vi "Splash.vi"(4 "warning sign":refnum<vi>, 5 "Cluster control array":refnum<vi>[](array[refnum])=[refnum, refnum, refnum], 6 "Firmware :":refnum<vi>, 7 "Pressure:":refnum<vi>, 8 "error in (no error)":errorcluster, 10 "Init Ref":T1, 11 "Stop":refnum<vi>) -> (0 "error out":errorcluster)   [LabVIEW 2018]
uses:
  PublicSubVI/Class/FileManager/FM/ctl/_PC_Pub_FM ctrlFileRefnumEnum.ctl
  PublicSubVI/Ctl/RegistyFunc.ctl
  <vilib>/Utility/error.llb/Error Cluster From Error Code.vi
  <vilib>/ErrorRing/Error Ring.xnode
  PublicSubVI/Class/SigInfo/SigInfo.lvclass
  PublicSubVI/Class/Sig2MS/Sig2MS.lvclass
panel:
  out "Status String Display":string
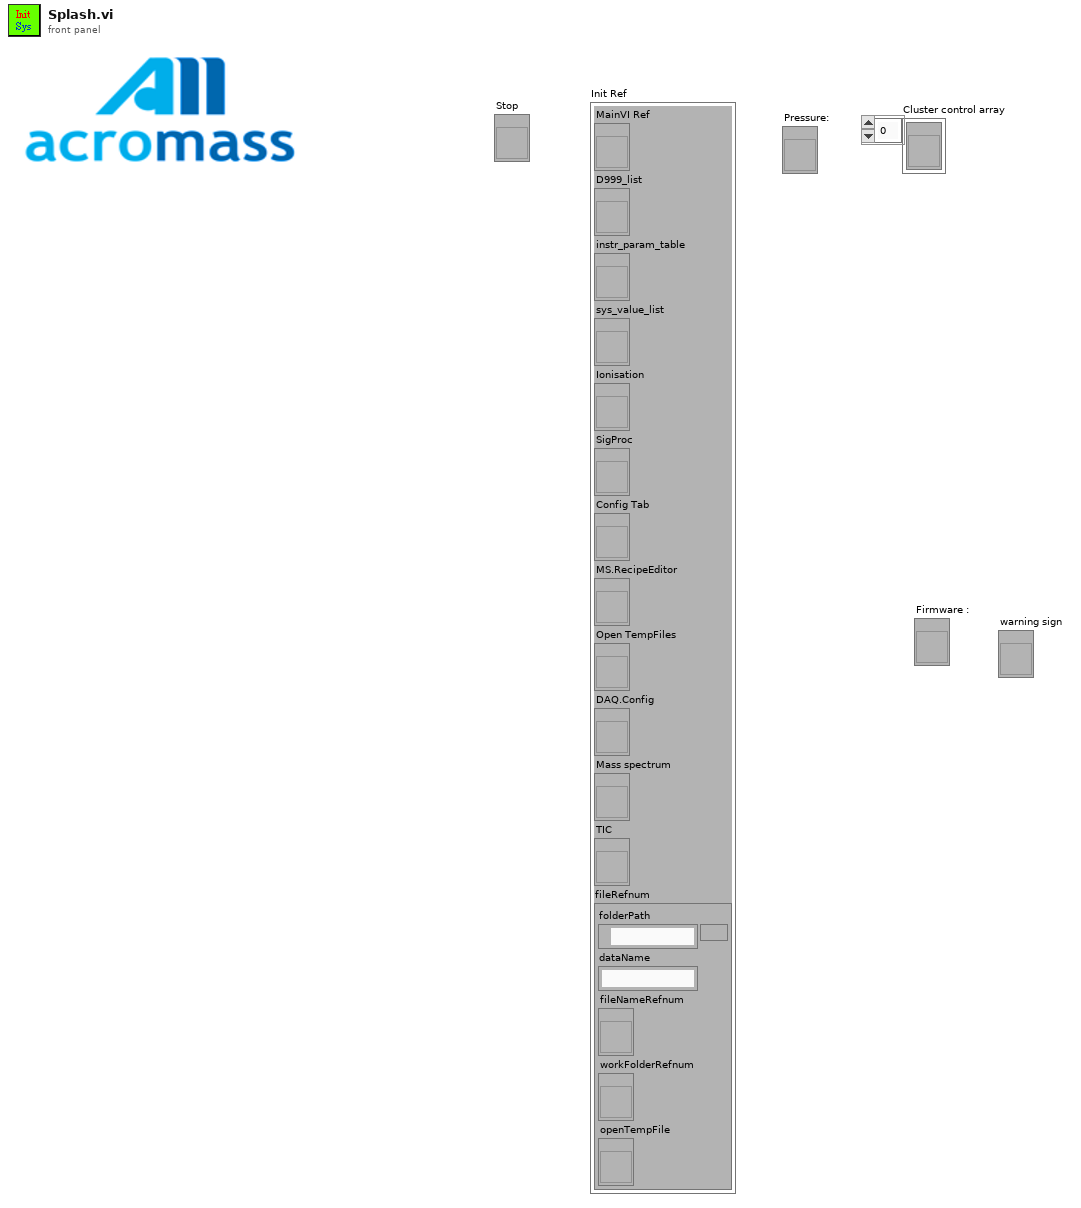
[diagram p1: front panel]
types:
  T1 = cluster{"MainVI Ref":refnum<vi>, "D999_list":refnum<vi>, "instr_param_table":refnum<vi>, "sys_value_list":refnum<vi>, "Ionisation":refnum<vi>, "SigProc":refnum<vi>, "Config Tab":refnum<vi>, "MS.RecipeEditor":refnum<vi>, "Open TempFiles":refnum<vi>, "DAQ.Config":refnum<vi>, "Mass spectrum":refnum<vi>, "TIC":refnum<vi>, "fileRefnum":cluster{"folderPath":path, "dataName":string, "fileNameRefnum":refnum<vi>, "workFolderRefnum":refnum<vi>, "openTempFile":refnum<vi>}}
  T2 = enum16{"init", "writeState", "readState", "close"}
  T3 = enum16{"init", "loadScript", "newScript", "runScript", "close"}
  T4 = typedef "RegistyFunc.ctl" = enum16{"None", "FileAutoSave", "FileNoise", "FileSN", "ExeStatu", "WorkFolderPath", "MethodPath", "AVGItem", "LoopItem", "AutoRun", "BGColor", "LineColor", "LineWidth", "XGrid", "YGrid", "DeviceRefnum"}
  T5 = typedef "_PC_Pub_FM ctrlFileRefnumEnum.ctl" = enum16{"init", "checkFileName", "updFileName", "updWorkFolder", "updDataItems", "addNewFileName", "addSerialNum"}
  T6 = cluster{"This VI":refnum<vi>, "Config Tab":refnum<vi>, "D999_value":refnum<vi>, "Parameter":refnum<vi>, "System":refnum<vi>}
  T7 = enum8{"Enabled", "Disabled", "Disabled and Grayed Out"}
  T8 = enum32{"Invalid", "Default", "Floating", "Floating/Auto-Hide", "Modal"}
  T9 = cluster{"folderPath":path, "dataName":string, "fileNameRefnum":refnum<vi>, "workFolderRefnum":refnum<vi>, "openTempFile":refnum<vi>}
  T10 = cluster{"config tab":refnum<vi>, "d999 value list":refnum<vi>, "param table":refnum<vi>, "sys_value list":refnum<vi>}
  T11 = cluster{"Pressure chart":refnum<vi>, "Turbo pump status":refnum<vi>, "Turbo speed":refnum<vi>, "Turbo power":refnum<vi>, "RT Resource":refnum<vi>, "Pressure realtime":refnum<vi>, "Voltage":refnum<vi>, "Pressure string":refnum<vi>}
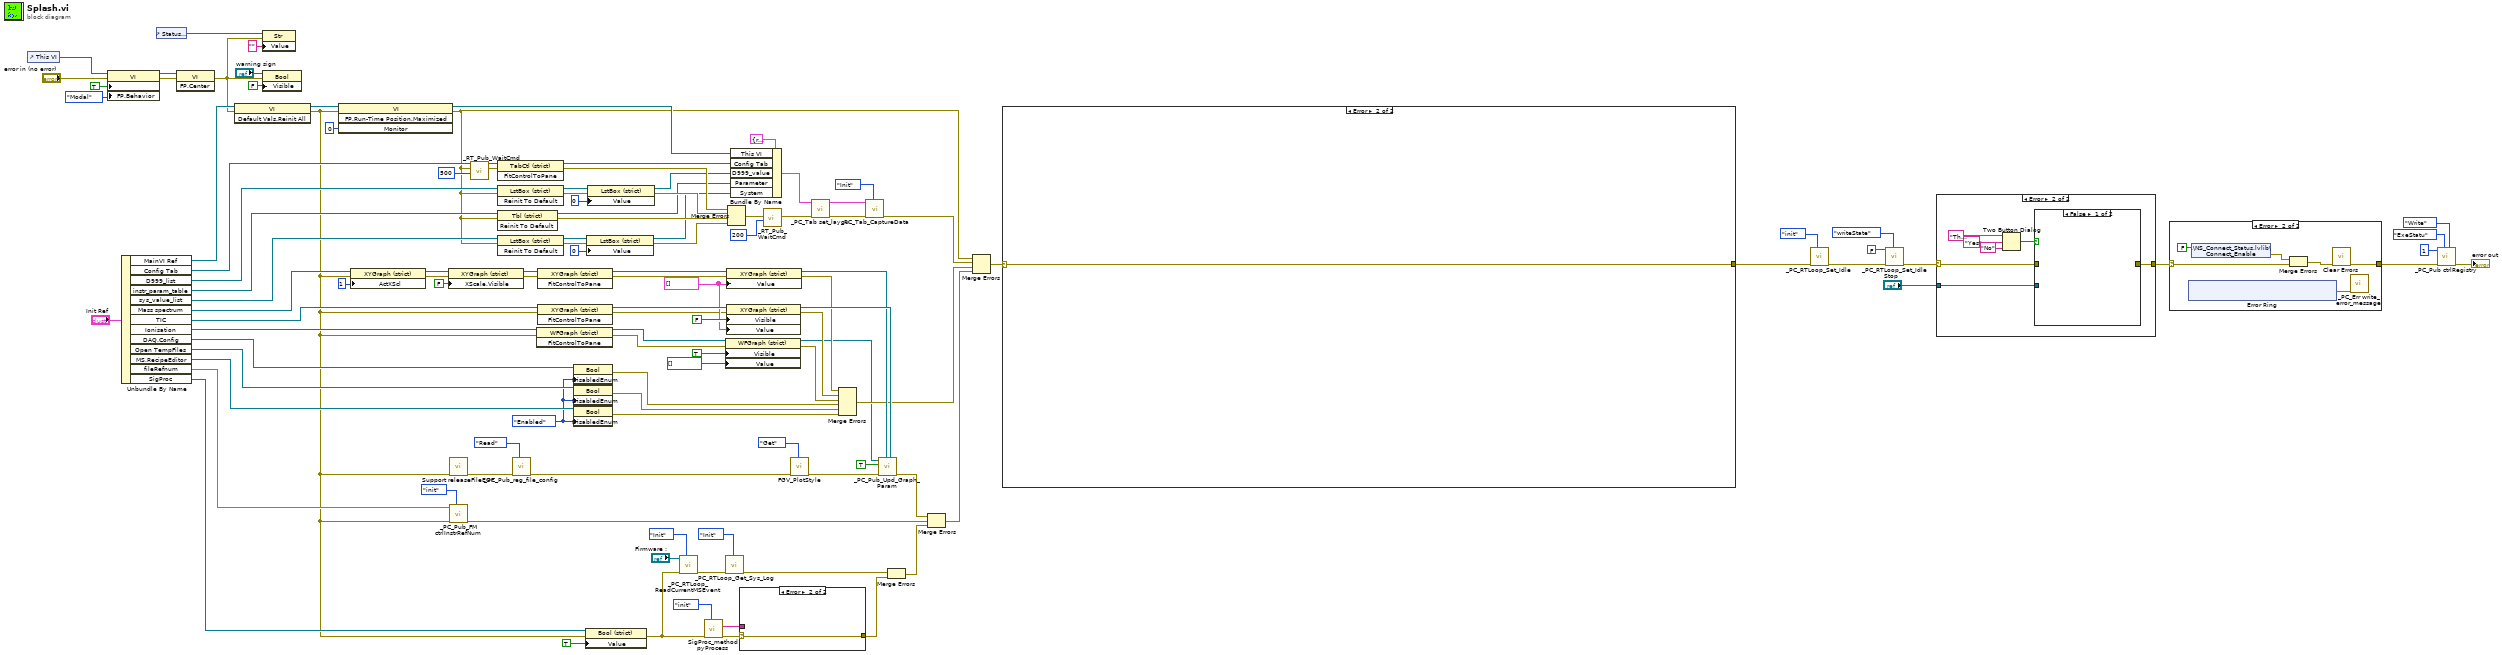
[diagram p0: block diagram]
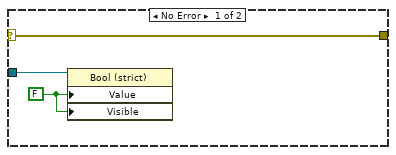
[diagram p2: hidden frame]
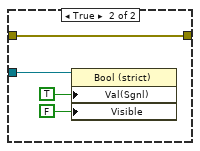
[diagram p3: hidden frame]
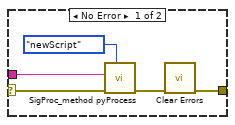
[diagram p4: hidden frame]
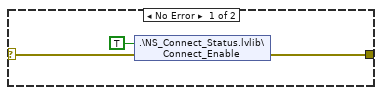
[diagram p5: hidden frame]
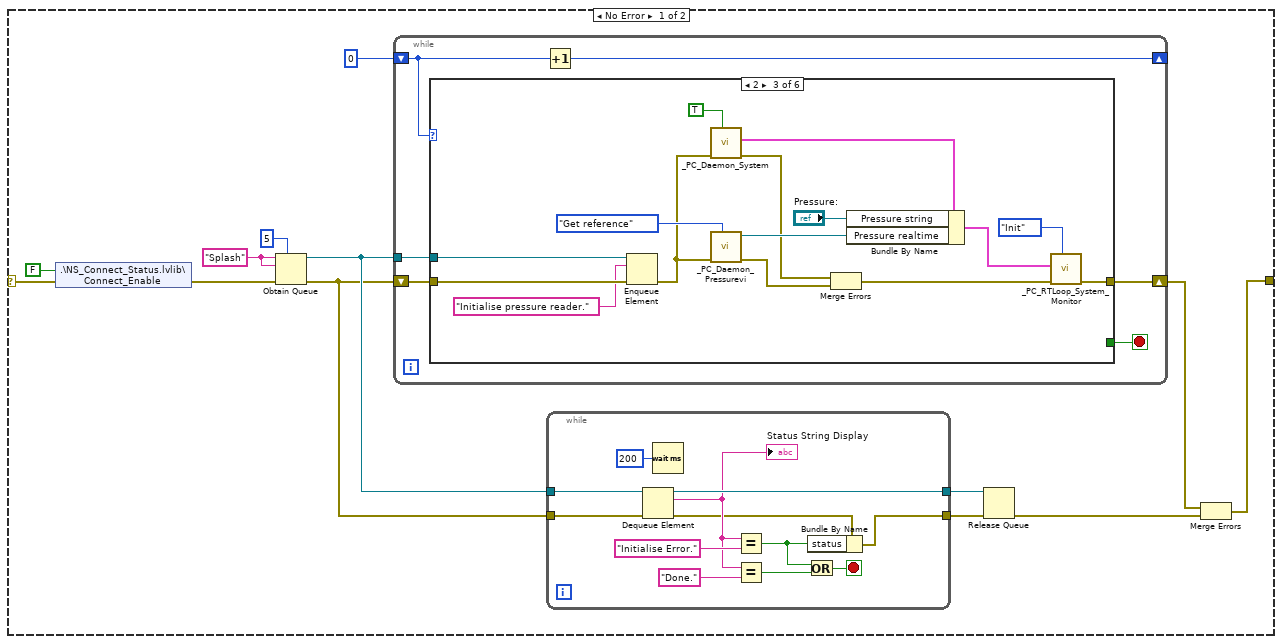
[diagram p6: hidden frame]
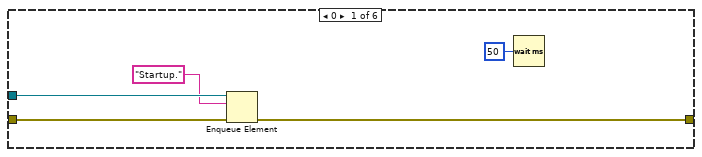
[diagram p7: hidden frame]
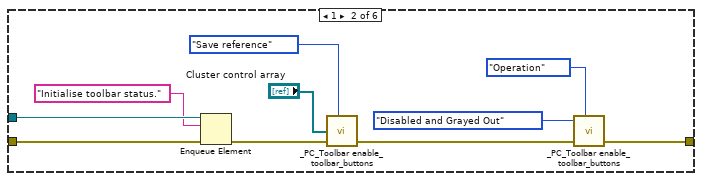
[diagram p8: hidden frame]
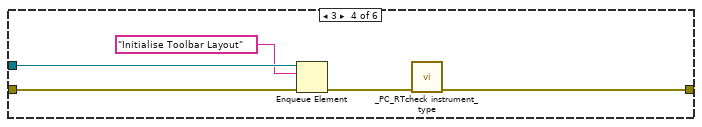
[diagram p9: hidden frame]
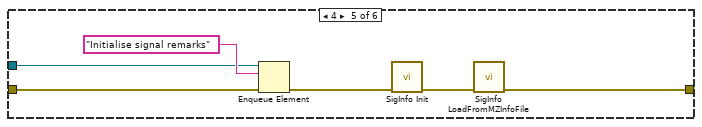
[diagram p10: hidden frame]
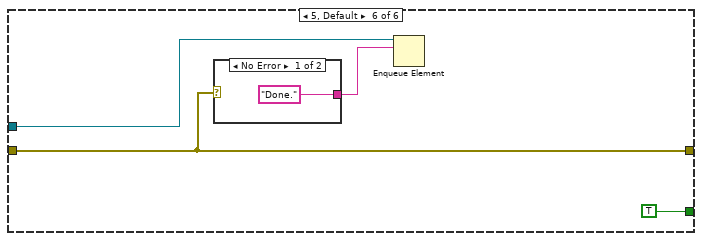
[diagram p11: hidden frame]
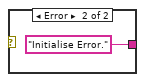
[diagram p12: hidden frame]
diagram:
  w95 = T7."Enabled" ("Disabled")
  w105 = cluster{"X":dbl[], "Y":sgl[]}[] [] ("appended array")
  n1 = control-ref of="This VI"() -> (w104:refnum<vi>)
  n2 = property class="VI"(reference=w104, error in="error in (no error)", "Front Panel.IsFrontmost"=TRUE, "FP.Behavior"=T8."Modal" ("Front Panel Window:Behavior")) -> (reference out=w100:refnum<vi>, error out=w99:errorcluster)
  n3 = Unbundle By Name("Init Ref") -> ("MainVI Ref"=w66:refnum<vi>, "Config Tab"=w65:refnum<vi>, "D999_list"=w64:refnum<vi>, "instr_param_table"=w63:refnum<vi>, "sys_value_list"=w62:refnum<vi>, "Mass spectrum"=w27:refnum<vi>, "TIC"=w115:refnum<vi>, "Ionisation"=w114:refnum<vi>, "DAQ.Config"=w98:refnum<vi>, "Open TempFiles"=w97:refnum<vi>, "MS.RecipeEditor"=w96:refnum<vi>, "fileRefnum"=w41:T9, "SigProc"=w69:refnum<vi>)
  n4 = control-ref of="Status String Display"() -> (w13:refnum<vi>)
  n5 = invoke class="VI" method="FP.Center"(reference=w100, error in=w99) -> (error out=w12:errorcluster)  [unwired: 1 in, 2 out]
  n6 = invoke class="VI" method="Default Vals.Reinit All"(reference=w66, error in=w12) -> (reference out=w84:refnum<vi>, error out=w10:errorcluster)  [unwired: 1 in, 1 out]
  n7 = property class="Str"(reference=w13, error in=w12, "Value"="") -> ()  [unwired: 2 out]
  n8 = property class="Bool"(reference="warning sign", error in=w12, "Visible"=FALSE) -> ()  [unwired: 2 out]
  n9 = invoke class="VI" method="FP.Run-Time Position.Maximized"(reference=w84, error in=w10, "Monitor"=i16 0) -> (reference out=w53:refnum<vi>, error out=w43:errorcluster)  [unwired: 1 in, 2 out]
  n10 = property class="XYGraph (strict)"(reference=w27, error in=w10, "ActXScl"=1 ("Active X Scale")) -> (reference out=w32:refnum<vi>, error out=w33:errorcluster)
  n11 = property class="XYGraph (strict)"(reference=w32, error in=w33, "XScale.Visible"=FALSE ("X Scale.Visible")) -> (reference out=w28:refnum<vi>, error out=w29:errorcluster)
  n12 = call "Support releaseFileEOF.vi"("error in (no error)"=w10) -> ("error out"=w26:errorcluster)  [unwired: 10 in]
  n13 = call "_PC_Pub_FM ctrlInstrRefNum.vi"("function"=_PC_Pub_FM_ctrlFileRefnumEnum."init", "error in (no error)"=w10, "Refnum"=w41) -> ("error out"=w40:errorcluster)  [unwired: 8 in]
  n14 = call "_RT_Pub_WaitCmd.vi"("milliseconds to wait"=u32 500, "error in (no error)"=w43) -> ("error out"=w71:errorcluster)  [unwired: 9 in]
  n15 = invoke class="TabCtl (strict)" method="FitControlToPane"(reference=w65, error in=w71) -> (reference out=w52:refnum<vi>, error out=w56:errorcluster)  [unwired: 1 in, 1 out]
  n16 = invoke class="LstBox (strict)" method="Reinit To Default"(reference=w64, error in=w43) -> (reference out=w108:refnum<vi>, error out=w94:errorcluster)  [unwired: 1 in, 1 out]
  n17 = invoke class="Tbl (strict)" method="Reinit To Default"(reference=w63, error in=w43) -> (reference out=w50:refnum<vi>, error out=w54:errorcluster)  [unwired: 1 in, 1 out]
  n18 = invoke class="LstBox (strict)" method="Reinit To Default"(reference=w62, error in=w43) -> (reference out=w60:refnum<vi>, error out=w59:errorcluster)  [unwired: 1 in, 1 out]
  n19 = call "_PC_Pub_reg_file_config.vi"("func"=enum16{"None", "Write", "Read"}."Read", "error in (no error)"=w26) -> ("error out"=w21:errorcluster)  [unwired: 3 in, 3 out]
  n20 = invoke class="WFGraph (strict)" method="FitControlToPane"(reference=w114, error in=w10) -> (reference out=w112:refnum<vi>, error out=w91:errorcluster)  [unwired: 1 in, 1 out]
  n21 = invoke class="XYGraph (strict)" method="FitControlToPane"(reference=w28, error in=w29) -> (reference out=w111:refnum<vi>, error out=w93:errorcluster)  [unwired: 1 in, 1 out]
  n22 = invoke class="XYGraph (strict)" method="FitControlToPane"(reference=w115, error in=w10) -> (reference out=w113:refnum<vi>, error out=w92:errorcluster)  [unwired: 1 in, 1 out]
  n23 = property class="Bool"(reference=w98, "DisabledEnum"=w95) -> (error out=w87:errorcluster)  [unwired: 1 in, 1 out]
  n24 = property class="Bool"(reference=w97, "DisabledEnum"=w95) -> (error out=w86:errorcluster)  [unwired: 1 in, 1 out]
  n25 = property class="Bool"(reference=w96, "DisabledEnum"=w95) -> (error out=w85:errorcluster)  [unwired: 1 in, 1 out]
  n26 = property class="Bool (strict)"(reference=w69, error in=w10, "Value"=TRUE) -> (error out=w18:errorcluster)  [unwired: 1 out]
  n27 = property class="LstBox (strict)"(reference=w60, error in=w59, "Value"=0) -> (reference out=w25:refnum<vi>, error out=w24:errorcluster)
  n28 = property class="LstBox (strict)"(reference=w108, error in=w94, "Value"=0) -> (reference out=w51:refnum<vi>, error out=w55:errorcluster)
  n29 = call "_PC_RTLoop_ReadCurrentMSEvent.vi"("Function"=enum16{"Init", "Get Data", "Close"}."Init", "error in (no error)"=w18, "Firmware string refin"="Firmware :") -> ("error out"=w34:errorcluster)  [unwired: 8 in]
  n30 = call "SigProc_method pyProcess.vi"("func"=T3."init", "error in (no error)"=w18) -> ("error out"=w17:errorcluster, "pyCode"=w19:string)  [unwired: 6 in, 2 out]
  n31 = property on="Property Node" class="WFGraph (strict)"(reference=w112, error in=w91, "Visible"=TRUE, "Value"=waveform(dbl)[] [] ("Ionisation")) -> (reference out=w22:refnum<vi>, error out=w88:errorcluster)
  n32 = call "_PC_RTLoop_Get_Sys_Log.vi"("Function"=enum16{"Init", "Get Data", "Close"}."Init", "error in (no error)"=w34) -> ("error out"=w16:errorcluster)  [unwired: 9 in]
  n33 = property on="Property Node" class="XYGraph (strict)"(reference=w113, error in=w92, "Visible"=FALSE, "Value"=w105) -> (reference out=w106:refnum<vi>, error out=w89:errorcluster)
  n34 = property on="Property Node" class="XYGraph (strict)"(reference=w111, error in=w93, "Value"=w105) -> (reference out=w79:refnum<vi>, error out=w90:errorcluster)
  n35 = Merge Errors(w56, w55, w54, w24) -> (w47:errorcluster)
  n36 = Bundle By Name(cluster=T6 {"This VI"=refnum, "Config Tab"=refnum, "D999_value"=refnum, "Parameter"=refnum, "System"=refnum} ("input cluster"), "This VI"=w53, "Config Tab"=w52, "D999_value"=w51, "Parameter"=w50, "System"=w25) -> (w49:T6)
  n37 = case shown="Error" w17 {
    selector: w17 -> [w121 w124]
    tunnel: w19 -> [w122 _]
    tunnel: [w119 w124] -> w15
    frame No Error {
      n38 = call "SigProc_method pyProcess.vi"("func"=T3."newScript", "error in (no error)"=w121, "newScriptCode"=w122) -> ("error out"=w120:errorcluster)  [unwired: 5 in, 3 out]
      n39 = call <vilib>:"Clear Errors.vi"("error in (no error)"=w120) -> ("error out"=w119:errorcluster)  [unwired: 5 in, 1 out]
    }
    frame Error {
    }
  }
  n40 = call "_RT_Pub_WaitCmd.vi"("milliseconds to wait"=u32 200, "error in (no error)"=w47) -> ("error out"=w46:errorcluster)  [unwired: 9 in]
  n41 = call "FGV_PlotStyle.vi"("Function"=enum16{"Set", "Get"}."Get", "error in (no error)"=w21) -> ("error out"=w81:errorcluster)  [unwired: 8 in, 1 out]
  n42 = call "_PC_Tab set_layou.vi"("error in (no error)"=w46, "input cluster"=w49) -> ("error out"=w57:errorcluster, "tab ctrl refnums"=w58:T10)  [unwired: 8 in]
  n43 = Merge Errors(w90, w89, w88, w87, w86, w85) -> (w76:errorcluster)
  n44 = call "_PC_Tab_CaptureData.vi"("Function"=enum16{"Init", "Get Data", "Update", "Close"}."Init", "error in (no error)"=w57, "tab ctrl refnums"=w58) -> ("error out"=w75:errorcluster)  [unwired: 8 in]
  n45 = call "_PC_Pub_Upd_Graph_Param.vi"("TIC"=w106, "Mass spectrum"=w79, "error in (no error)"=w81, "Init?(F)"=TRUE, "Ionisation"=w22) -> ("error out"=w78:errorcluster)  [unwired: 6 in]
  n46 = Merge Errors(w16, w15) -> (w14:errorcluster)
  n47 = Merge Errors(w78, w40, w14) -> (w77:errorcluster)
  n48 = Merge Errors(w43, w75, w76, w77) -> (w110:errorcluster)
  n49 = case shown="Error" w110 {
    selector: w110 -> [w130 w203]
    tunnel: [w126 w203] -> w9
    frame No Error {
      w136 = "Splash" ("name (unnamed)")
      n50 = shared-variable ".\\NS_Connect_Status.lvlib\\Connect_Enable"(FALSE ("Connect_Enable"), error in=w130) -> (error out=w127:errorcluster)
      n51 = Obtain Queue(max queue size (-1, unlimited)=5, name (unnamed)=w136, element data type=w136, error in (no error)=w127) -> (queue out=w135:refnum<queue>, error out=w134:errorcluster)  [unwired: 1 in, 1 out]
      n52 = while {
        tunnel: w135 -> [w153]
        shift-right: [w152] -> _
        shift-left: u8 0 -> [w155]
        shift-right: [w150] -> w129
        shift-left: w134 -> [w154]
        stop <- w151 stop-if-true
        n53 = case shown="2" w155 {
          tunnel: w154 -> [w158 w162 w184 w189 w192 w197]
          tunnel: [w157 w165 w172 w186 w195 w197] -> w150
          tunnel: w153 -> [w160 w164 w183 w190 w193 w199]
          tunnel: [_ _ _ _ _ TRUE] -> w151
          frame 0 {
            n54 = Enqueue Element(queue=w160, element="Startup." ("string in"), error in (no error)=w158) -> (error out=w157:errorcluster)  [unwired: 1 in, 2 out]
            n55 = Wait (ms)(milliseconds to wait=u32 50) -> ()  [unwired: 1 out]
          }
          frame 1 {
            n56 = Enqueue Element(queue=w164, element="Initialise toolbar status." ("string in"), error in (no error)=w162) -> (error out=w161:errorcluster)  [unwired: 1 in, 2 out]
            n57 = call "_PC_Toolbar enable_toolbar_buttons.vi"("Function"=enum16{"Save reference", "Operation"}."Save reference", "Cluster control array"="Cluster control array", "error in (no error)"=w161) -> ("error out"=w168:errorcluster)  [unwired: 6 in]
            n58 = call "_PC_Toolbar enable_toolbar_buttons.vi"("Disabled"=T7."Disabled and Grayed Out", "Function"=enum16{"Save reference", "Operation"}."Operation", "error in (no error)"=w168) -> ("error out"=w165:errorcluster)  [unwired: 6 in]
          }
          frame 2 {
            n59 = Enqueue Element(queue=w183, element="Initialise pressure reader." ("string in"), error in (no error)=w184) -> (error out=w178:errorcluster)  [unwired: 1 in, 2 out]
            n60 = call "_PC_Daemon_System.vi"("GetRef? ( F )"=TRUE, "error in (no error)"=w178) -> ("error out"=w177:errorcluster, "Instrument Parmeter"=w180:T11)  [unwired: 8 in]
            n61 = call "_PC_Daemon_Pressurevi.vi"("Function"=enum16{"Get reference", "Show graph"}."Get reference", "error in (no error)"=w178) -> ("error out"=w176:errorcluster, "XY Graph"=w179:refnum<vi>)  [unwired: 8 in]
            n62 = Merge Errors(w177, w176) -> (w173:errorcluster)
            n63 = Bundle By Name(cluster=w180, "Pressure string"="Pressure:", "Pressure realtime"=w179) -> (w174:T11)
            n64 = call "_PC_RTLoop_System_Monitor.vi"("Function"=enum16{"Init", "Get Data", "Close"}."Init", "error in (no error)"=w173, "Instrument Parmeter"=w174) -> ("error out"=w172:errorcluster)  [unwired: 8 in]
          }
          frame 3 {
            n65 = Enqueue Element(queue=w190, element="Initialise Toolbar Layout" ("set string"), error in (no error)=w189) -> (error out=w187:errorcluster)  [unwired: 1 in, 2 out]
            n66 = call "_PC_RTcheck instrument_type.vi"("error in (no error)"=w187) -> ("error out"=w186:errorcluster)  [unwired: 10 in]
          }
          frame 4 {
            n67 = Enqueue Element(queue=w193, element="Initialise signal remarks" ("set string"), error in (no error)=w192) -> (error out=w191:errorcluster)  [unwired: 1 in, 2 out]
            n68 = call "SigInfo Init.vi"("error in (no error)"=w191) -> ("error out"=w196:errorcluster)  [unwired: 9 in, 1 out]
            n69 = call "SigInfo LoadFromMZInfoFile.vi"("error in (no error)"=w196) -> ("error out"=w195:errorcluster)  [unwired: 9 in, 1 out]
          }
          frame 5, Default {
            n70 = case shown="No Error" w197 {
              tunnel: ["Done." ("string in") "Initialise Error." ("set string")] -> w198
              frame No Error {
              }
              frame Error {
              }
            }
            n71 = Enqueue Element(queue=w199, element=w198) -> ()  [unwired: 2 in, 3 out]
          }
        }
        n72 = Increment(x=w155) -> (x+1=w152:u8)
      }
      n73 = while {
        tunnel: w135 -> [w149]
        tunnel: w134 -> [w148]
        tunnel: [w144] -> w132
        tunnel: [w138] -> w125
        stop <- w145 stop-if-true
        n74 = Dequeue Element(queue=w149, error in (no error)=w148) -> (queue out=w144:refnum<queue>, element=w143:string, error out=w140:errorcluster)  [unwired: 1 in, 1 out]
        "Status String Display" <- w143
        n75 = Wait (ms)(milliseconds to wait=u32 200) -> ()  [unwired: 1 out]
        n76 = Equal?(x=w143, y="Initialise Error.") -> (x = y?=w139:bool)
        n77 = Equal?(x=w143, y="Done.") -> (x = y?=w141:bool)
        n78 = Or(x=w139, y=w141) -> (x .or. y?=w145:bool)
        n79 = Bundle By Name(cluster=w140, "status"=w139) -> (w138:errorcluster)
      }
      n80 = Release Queue(queue=w132, error in (no error)=w125) -> (error out=w128:errorcluster)  [unwired: 1 in, 2 out]
      n81 = Merge Errors(w129, w128) -> (w126:errorcluster)
    }
    frame Error {
    }
  }
  n82 = call "_PC_RTLoop_Set_Idle.vi"("Function"=T2."init", "error in (no error)"=w9) -> ("error out"=w5:errorcluster)  [unwired: 8 in, 1 out]
  n83 = call "_PC_RTLoop_Set_Idle.vi"("Function"=T2."writeState", "error in (no error)"=w5, "exe_state"=FALSE ("exe_statu")) -> ("error out"=w4:errorcluster)  [unwired: 7 in, 1 out]
  n84 = case shown="Error" w4 {
    selector: w4 -> [w204 w209]
    tunnel: "Stop" -> [w205 w207]
    tunnel: [w204 w208] -> w2
    frame No Error {
      w206 = FALSE ("Value")
      n85 = property class="Bool (strict)"(reference=w205, "Value"=w206, "Visible"=w206) -> ()  [unwired: 1 in, 2 out]
    }
    frame Error {
      n86 = Two Button Dialog(message="The system can not detect, do you want to close this software?", 1:"No" ("F button name (\"Cancel\")"), 2:"Yes" ("T button name (\"OK\")")) -> (T button?=w210:bool)
      n87 = case shown="False" w210 {
        tunnel: w209 -> [_ w217]
        tunnel: [_ w217] -> w208
        tunnel: w207 -> [_ w215]
        frame False {
        }
        frame True {
          n88 = property class="Bool (strict)"(reference=w215, "Val(Sgnl)"=TRUE ("Value"), "Visible"=FALSE ("Value")) -> ()  [unwired: 1 in, 2 out]
        }
      }
    }
  }
  n89 = case shown="Error" w2 {
    selector: w2 -> [w219 w223]
    tunnel: [w218 w221] -> w1
    frame No Error {
      n90 = shared-variable ".\\NS_Connect_Status.lvlib\\Connect_Enable"(TRUE ("Connect_Enable"), error in=w219) -> (error out=w218:errorcluster)
    }
    frame Error {
      n91 = xnode "Error Ring"() -> ("error out"=w226:errorcluster)
      n92 = shared-variable ".\\NS_Connect_Status.lvlib\\Connect_Enable"(FALSE ("Connect_Enable")) -> (error out=w224:errorcluster)  [unwired: 1 in]
      n93 = Merge Errors(w224, w223) -> (w222:errorcluster)
      n94 = call <vilib>:"Clear Errors.vi"("error in (no error)"=w222) -> ("error out"=w221:errorcluster)  [unwired: 5 in, 1 out]
      n95 = call "_PC_Err write_error_message.vi"("error in"=w226) -> ()  [unwired: 10 in, 1 out]
    }
  }
  n96 = call "_PC_Pub ctrlRegistry.vi"("type"=enum16{"None", "Write", "Read"}."Write", "function"=RegistyFunc."ExeStatu", "error in (no error)"=w1, "write value"=1) -> ("error out"=→"error out":errorcluster)  [unwired: 4 in, 3 out]
